vi "Command Drive Path.vi"(2 "All Robot Commands In":T1, 3 "Startup":bool, 4 "Cmd Parameter 4":string, 5 "Cmd Parameter 3":dbl, 6 "Cmd Parameter 2":dbl, 7 "Cmd Parameter 1":dbl) -> (0 "All Robot Commands Out":T1, 1 "Completed":bool)   [LabVIEW 2016]
uses:
  Subsystems/All Robot Commands.ctl
  Subsystems/Drive and Climb SS/Drive + Climb Commands 2017.ctl
  Subsystems/Gear Delivery SS/Gear Delivery Commands.ctl
  Subsystems/Conveyor and Shooter SS/Conveyor and Shooter Commands.ctl
  Subsystems/Ball Intake SS/Ball Intake Commands.ctl
  Command Execution State.ctl
  <vilib>/Rock Robotics/WPI/ThirdParty/CanMotor/TalonSRX/WPI_CANTalonSRX_APIControlMode.ctl
  Global Variables/Drive Path Logging Data.vi
  Global Variables/MotionProfile.vi
  Global Variables/Refnum Names.vi
  Global Variables/Drive Path Calibrations.vi
panel:
  out "Right F":dbl
  out "Right D":dbl
  out "Right I":dbl
  out "Right P":dbl
  out "Left F":dbl
  out "Left D":dbl
  out "Left I":dbl
  out "Left P":dbl
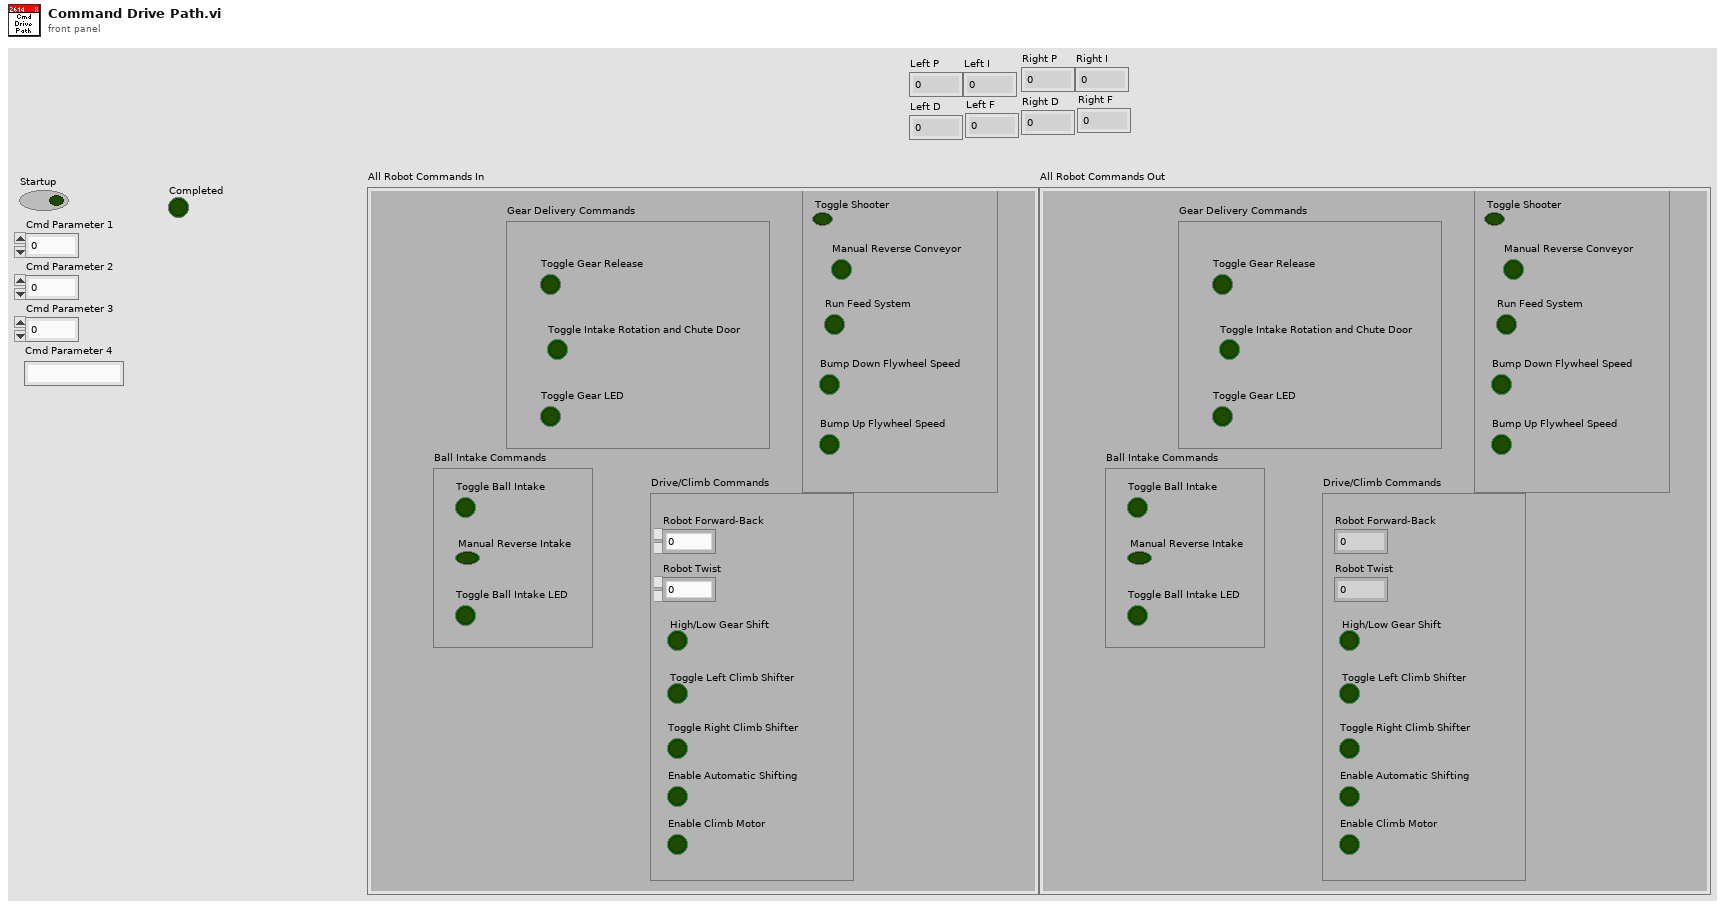
[diagram p1: front panel]
types:
  T1 = typedef "All Robot Commands.ctl" = cluster{"Drive/Climb Commands":T2, "Gear Delivery Commands":T3, "Shooter and Conveyor Commands":T4, "Ball Intake Commands":T5}
  T2 = typedef "Drive + Climb Commands 2017.ctl" = cluster{"Robot Forward-Back":dbl, "Robot Twist":dbl, "High/Low Gear Shift":bool, "Toggle Left Climb Shifter":bool, "Toggle Right Climb Shifter":bool, "Enable Automatic Shifting":bool, "Enable Climb Motor ":bool}
  T3 = typedef "Gear Delivery Commands.ctl" = cluster{"Toggle Gear Release":bool, "Toggle Intake Rotation and Chute Door":bool, "Toggle Gear LED":bool}
  T4 = typedef "Conveyor and Shooter Commands.ctl" = cluster{"Toggle Shooter":bool, "Manual Reverse Conveyor":bool, "Run Feed System":bool, "Bump Down Flywheel Speed":bool, "Bump Up Flywheel Speed":bool}
  T5 = typedef "Ball Intake Commands.ctl" = cluster{"Toggle Ball Intake":bool, "Manual Reverse Intake":bool, "Toggle Ball Intake LED":bool}
  T6 = typedef "Command Execution State.ctl" = enum16{"Initialize", "Execute", "Finish"}
  T7 = typedef "WPI_CANTalonSRX_APIControlMode.ctl" = enum8{"Percent VBus", "Speed", "Position", "Slave", "Unchanged / Invalid", "Voltage Compensation", "Current", "Motion Profile", "Motion Magic"}
  T8 = typedef "WPI_MotorControlDeviceRef.ctl" = cluster{"DeviceStatus":errorcluster, "Type":T9, "PWM":cluster{"PWM Channel":T10, "DeadBand":T11}, "CAN":cluster{"Device Number":u8, "SetOutput VI Ref":variant, "GetOutput VI Ref":variant, "Enable VI Ref":variant, "Disable VI Ref":variant, "Data":variant}, "Invert":bool}
  T9 = typedef "WPI_MotorControlType.ctl" = enum16{"PWM", "CAN"}
  T10 = typedef "FPGA_DIOPWMChannel.ctl" = enum8{"PWM 0", "PWM 1", "PWM 2", "PWM 3", "PWM 4", "PWM 5", "PWM 6", "PWM 7", "PWM 8", "PWM 9", "PWM MXP 0", "PWM MXP 1", "PWM MXP 2", "PWM MXP 3", "PWM MXP 4", "PWM MXP 5", "PWM MXP 6", "PWM MXP 7", "PWM MXP 8", "PWM MXP 9", "Invalid"}
  T11 = typedef "WPI_PWMDeadband.ctl" = cluster{"Name":string, "maxPositivePwm":i32, "minPositivePwm":i32, "centerPwm":i32, "maxNegativePwm":i32, "minNegativePwm":i32, "angularRange":u16}
  T12 = typedef "MotionProfile TypeDef.ctl" = cluster{"Left MP Array":dbl[][], "Left MP Index":dbl, "Semaphore":bool, "Right MP Array":dbl[][], "Right MP Index":dbl}
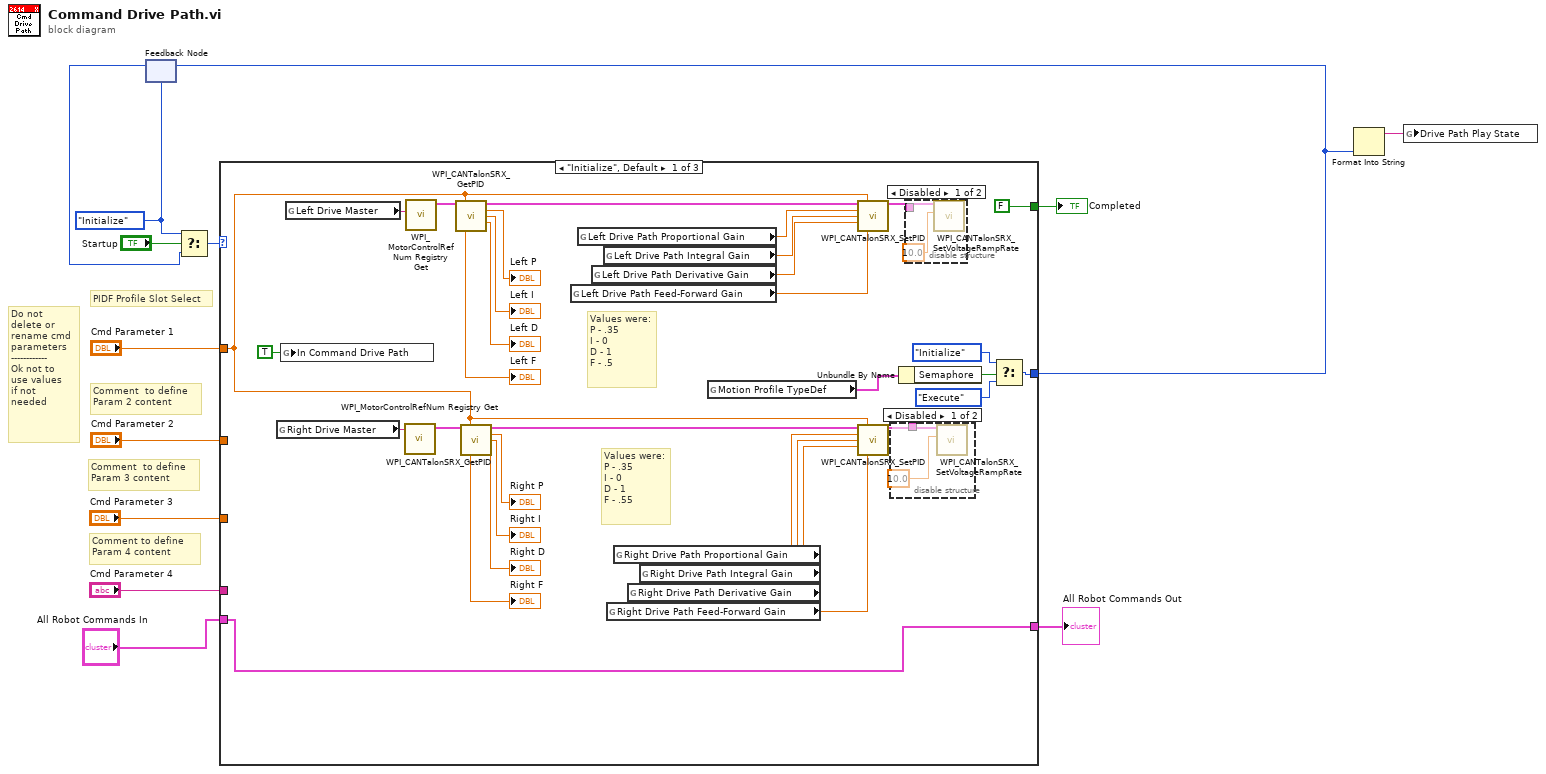
[diagram p0: block diagram]
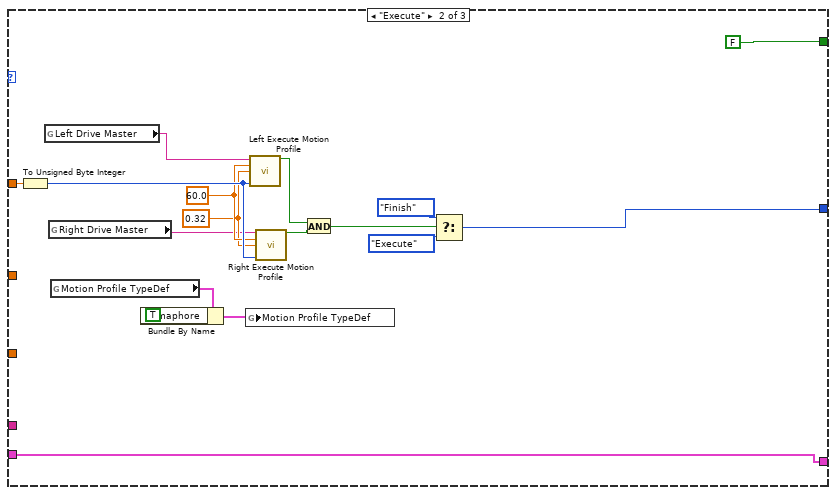
[diagram p4: hidden frame]
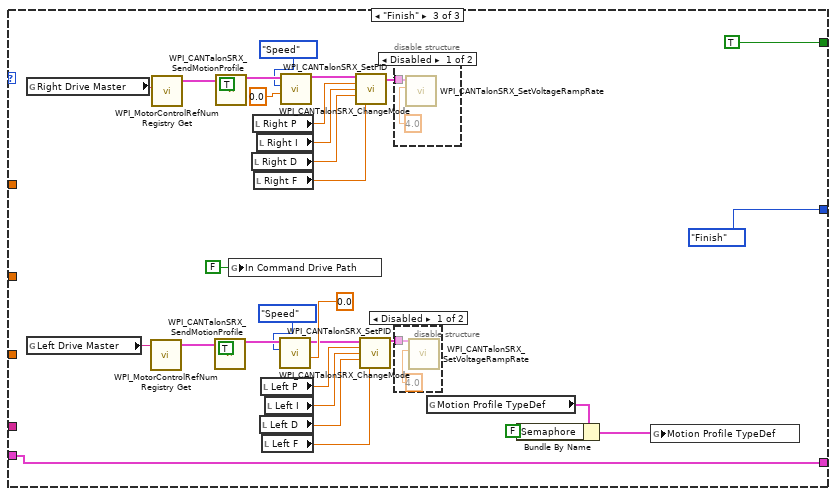
[diagram p5: hidden frame]
diagram:
  w5 = Command_Execution_State."Initialize" ("Play State")
  # "Comment to define \nParam 4 content"
  # "Comment  to define\nParam 3 content"
  # "Do not \ndelete or\nrename cmd\nparameters\n------------\nOk not to \nuse values\nif not \nneeded"
  # "Comment  to define\nParam 2 content"
  # "PIDF Profile Slot Select"
  n1 = feedback #1(w5) -> (w10:T6)
  n2 = Select(t=w5, s="Startup", f=w10) -> (s? t:f=w13:T6)
  n3 = case shown="\"Initialize\", Default" w13 {
    tunnel: [FALSE FALSE TRUE] -> w11
    tunnel: [w43 w64 Command_Execution_State."Finish" ("Play State")] -> w1
    tunnel: "Cmd Parameter 1" -> [w14 w60 _]
    tunnel: "Cmd Parameter 2" -> [_ _ _]
    tunnel: "Cmd Parameter 3" -> [_ _ _]
    tunnel: "Cmd Parameter 4" -> [_ _ _]
    tunnel: "All Robot Commands In" -> [w15 w51 w81]
    tunnel: [w15 w51 w81] -> w3
    frame "Initialize", Default {
      # "Values were:\nP - .35\nI - 0\nD - 1\nF - .55"
      # "Values were:\nP - .35\nI - 0\nD - 1\nF - .5"
      n4 = global read "Refnum Names.vi" "Right Drive Master"() -> (w40:string)
      n5 = global write "Drive Path Logging Data.vi" "In Command Drive Path"(TRUE ("In Command Drive Path")) -> ()
      n6 = global read "Refnum Names.vi" "Left Drive Master"() -> (w39:string)
      n7 = call <vilib>:"WPI_MotorControlRefNum Registry Get.vi"("refnum name"=w40) -> ("MotorControlDevRef"=w32:T8)  [unwired: 9 in, 1 out]
      n8 = call <vilib>:"WPI_MotorControlRefNum Registry Get.vi"("refnum name"=w39) -> ("MotorControlDevRef"=w38:T8)  [unwired: 9 in, 1 out]
      n9 = call <vilib>:"WPI_CANTalonSRX_GetPID.vi"("CAN Talon SRX Ref"=w38, "Parameter Slot"=w14) -> ("CAN Talon SRX Ref"=w31:T8, "P"=→"Left P":dbl, "I"=→"Left I":dbl, "D"=→"Left D":dbl, "F"=→"Left F":dbl)  [unwired: 6 in, 3 out]
      n10 = call <vilib>:"WPI_CANTalonSRX_GetPID.vi"("CAN Talon SRX Ref"=w32, "Parameter Slot"=w14) -> ("CAN Talon SRX Ref"=w27:T8, "P"=→"Right P":dbl, "I"=→"Right I":dbl, "D"=→"Right D":dbl, "F"=→"Right F":dbl)  [unwired: 6 in, 3 out]
      n11 = global read "Drive Path Calibrations.vi" "Left Drive Path Feed-Forward Gain"() -> (w26:dbl)
      n12 = global read "Drive Path Calibrations.vi" "Left Drive Path Proportional Gain"() -> (w23:dbl)
      n13 = global read "Drive Path Calibrations.vi" "Left Drive Path Derivative Gain"() -> (w25:dbl)
      n14 = global read "Drive Path Calibrations.vi" "Left Drive Path Integral Gain"() -> (w24:dbl)
      n15 = global read "Drive Path Calibrations.vi" "Right Drive Path Feed-Forward Gain"() -> (w19:dbl)
      n16 = global read "Drive Path Calibrations.vi" "Right Drive Path Proportional Gain"() -> (w22:dbl)
      n17 = global read "Drive Path Calibrations.vi" "Right Drive Path Derivative Gain"() -> (w20:dbl)
      n18 = global read "Drive Path Calibrations.vi" "Right Drive Path Integral Gain"() -> (w21:dbl)
      n19 = global read "MotionProfile.vi" "Motion Profile TypeDef"() -> (w42:T12)
      n20 = call <vilib>:"WPI_CANTalonSRX_SetPID.vi"("CAN Talon SRX Ref"=w31, "Parameter Slot"=w14, "P"=w23, "I"=w24, "D"=w25, "F"=w26) -> ("CAN Talon SRX Ref"=w18:T8)  [unwired: 8 in, 1 out]
      n21 = call <vilib>:"WPI_CANTalonSRX_SetPID.vi"("CAN Talon SRX Ref"=w27, "Parameter Slot"=w14, "P"=w22, "I"=w21, "D"=w20, "F"=w19) -> ("CAN Talon SRX Ref"=w17:T8)  [unwired: 8 in, 1 out]
      n22 = disable-structure shown="Disabled" {
        disable-tunnel: w17 -> [w48 _]
        frame Disabled {
          n23 = call <vilib>:"WPI_CANTalonSRX_SetVoltageRampRate.vi"("Throttle Ramp Rate (percent/s)"=10.0, "CAN Talon SRX Ref"=w48) -> ()  [unwired: 8 in, 2 out]
        }
        frame Enabled {
        }
      }
      n24 = Unbundle By Name(w42) -> ("Semaphore"=w41:bool)
      n25 = disable-structure shown="Disabled" {
        disable-tunnel: w18 -> [w50 _]
        frame Disabled {
          n26 = call <vilib>:"WPI_CANTalonSRX_SetVoltageRampRate.vi"("Throttle Ramp Rate (percent/s)"=10.0, "CAN Talon SRX Ref"=w50) -> ()  [unwired: 8 in, 2 out]
        }
        frame Enabled {
        }
      }
      n27 = Select(t=Command_Execution_State."Initialize" ("Play State"), s=w41, f=Command_Execution_State."Execute" ("Play State")) -> (s? t:f=w43:T6)
    }
    frame "Execute" {
      w57 = 0.32
      w58 = 60.0
      n28 = To Unsigned Byte Integer(number=w60) -> (unsigned 8bit integer=w59:u8)
      n29 = global read "Refnum Names.vi" "Left Drive Master"() -> (w53:string)
      n30 = global read "Refnum Names.vi" "Right Drive Master"() -> (w52:string)
      n31 = global read "MotionProfile.vi" "Motion Profile TypeDef"() -> (w56:T12)
      n32 = Bundle By Name(cluster=w56, "Semaphore"=TRUE) -> (w54:T12)
      n33 = global write "MotionProfile.vi" "Motion Profile TypeDef"(w54) -> ()
      n34 = call "Left Execute Motion Profile.vi"("Motor Name"=w53, "Time Conversion Factor"=w58, "Linear Conversion Factor"=w57, "PIDF Profile Slot Select"=w59) -> ("Complete"=w63:bool)  [unwired: 10 in, 1 out]
      n35 = call "Right Execute Motion Profile.vi"("Motor Name"=w52, "Time Conversion Factor"=w58, "Linear Conversion Factor"=w57, "PIDF Profile Slot Select"=w59) -> ("Complete"=w62:bool)  [unwired: 10 in, 1 out]
      n36 = And(x=w63, y=w62) -> (x .and. y?=w61:bool)
      n37 = Select(t=Command_Execution_State."Finish" ("Play State"), s=w61, f=Command_Execution_State."Execute" ("Play State")) -> (s? t:f=w64:T6)
    }
    frame "Finish" {
      n38 = global read "Refnum Names.vi" "Right Drive Master"() -> (w83:string)
      n39 = global read "Refnum Names.vi" "Left Drive Master"() -> (w82:string)
      n40 = call <vilib>:"WPI_MotorControlRefNum Registry Get.vi"("refnum name"=w82) -> ("MotorControlDevRef"=w92:T8)  [unwired: 9 in, 1 out]
      n41 = call <vilib>:"WPI_MotorControlRefNum Registry Get.vi"("refnum name"=w83) -> ("MotorControlDevRef"=w96:T8)  [unwired: 9 in, 1 out]
      n42 = call <vilib>:"WPI_CANTalonSRX_SendMotionProfile.vi"("CAN Talon SRX Ref"=w92, "Clear"=TRUE) -> ("CAN Talon SRX Ref Out"=w89:T8)  [unwired: 10 in, 3 out]
      n43 = call <vilib>:"WPI_CANTalonSRX_SendMotionProfile.vi"("CAN Talon SRX Ref"=w96, "Clear"=TRUE) -> ("CAN Talon SRX Ref Out"=w93:T8)  [unwired: 10 in, 3 out]
      n44 = global write "Drive Path Logging Data.vi" "In Command Drive Path"(FALSE ("In Command Drive Path")) -> ()
      n45 = local read "Right D"() -> (w77:dbl)
      n46 = local read "Right P"() -> (w79:dbl)
      n47 = local read "Right F"() -> (w76:dbl)
      n48 = local read "Right I"() -> (w78:dbl)
      n49 = local read "Left D"() -> (w72:dbl)
      n50 = local read "Left P"() -> (w74:dbl)
      n51 = local read "Left F"() -> (w71:dbl)
      n52 = local read "Left I"() -> (w73:dbl)
      n53 = call <vilib>:"WPI_CANTalonSRX_ChangeMode.vi"("Output"=0.0, "Control Mode"=WPI_CANTalonSRX_APIControlMode."Speed", "CAN Talon SRX Ref"=w89) -> ("CAN Talon SRX Ref"=w75:T8)  [unwired: 7 in, 1 out]
      n54 = call <vilib>:"WPI_CANTalonSRX_ChangeMode.vi"("Output"=0.0, "Control Mode"=WPI_CANTalonSRX_APIControlMode."Speed", "CAN Talon SRX Ref"=w93) -> ("CAN Talon SRX Ref"=w80:T8)  [unwired: 7 in, 1 out]
      n55 = call <vilib>:"WPI_CANTalonSRX_SetPID.vi"("CAN Talon SRX Ref"=w80, "P"=w79, "I"=w78, "D"=w77, "F"=w76) -> ("CAN Talon SRX Ref"=w70:T8)  [unwired: 9 in, 1 out]
      n56 = call <vilib>:"WPI_CANTalonSRX_SetPID.vi"("CAN Talon SRX Ref"=w75, "P"=w74, "I"=w73, "D"=w72, "F"=w71) -> ("CAN Talon SRX Ref"=w69:T8)  [unwired: 9 in, 1 out]
      n57 = disable-structure shown="Disabled" {
        disable-tunnel: w70 -> [w102 _]
        frame Disabled {
          n58 = call <vilib>:"WPI_CANTalonSRX_SetVoltageRampRate.vi"("Throttle Ramp Rate (percent/s)"=4.0, "CAN Talon SRX Ref"=w102) -> ()  [unwired: 8 in, 2 out]
        }
        frame Enabled {
        }
      }
      n59 = disable-structure shown="Disabled" {
        disable-tunnel: w69 -> [w100 _]
        frame Disabled {
          n60 = call <vilib>:"WPI_CANTalonSRX_SetVoltageRampRate.vi"("Throttle Ramp Rate (percent/s)"=4.0, "CAN Talon SRX Ref"=w100) -> ()  [unwired: 8 in, 2 out]
        }
        frame Enabled {
        }
      }
      n61 = global read "MotionProfile.vi" "Motion Profile TypeDef"() -> (w86:T12)
      n62 = Bundle By Name(cluster=w86, "Semaphore"=FALSE) -> (w84:T12)
      n63 = global write "MotionProfile.vi" "Motion Profile TypeDef"(w84) -> ()
    }
  }
  "Completed" <- w11
  "All Robot Commands Out" <- w3
  n64 = feedback-in #1(w1) -> ()
  n65 = Format Into String(w1) -> (resulting string=w2:string)  [unwired: 3 in, 1 out]
  n66 = global write "Drive Path Logging Data.vi" "Drive Path Play State"(w2) -> ()
